vi "rotation_to_euler.vi"(11 "Rotation":T1) -> (3 "Theta XYZ":dbl[](array[numeric]))   [LabVIEW 2013]
uses:
  <vilib>/Analysis/Matrix/Datatypes/RealMatrix.ctl
  <vilib>/Analysis/Matrix/NI_Matrix.lvlib
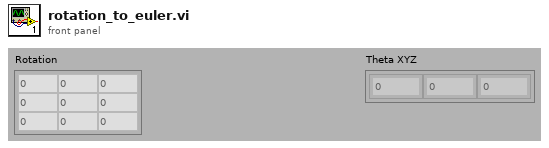
[diagram p1: front panel]
types:
  T1 = typedef "NI_Matrix.lvlib/RealMatrix.ctl" = dbl[][]
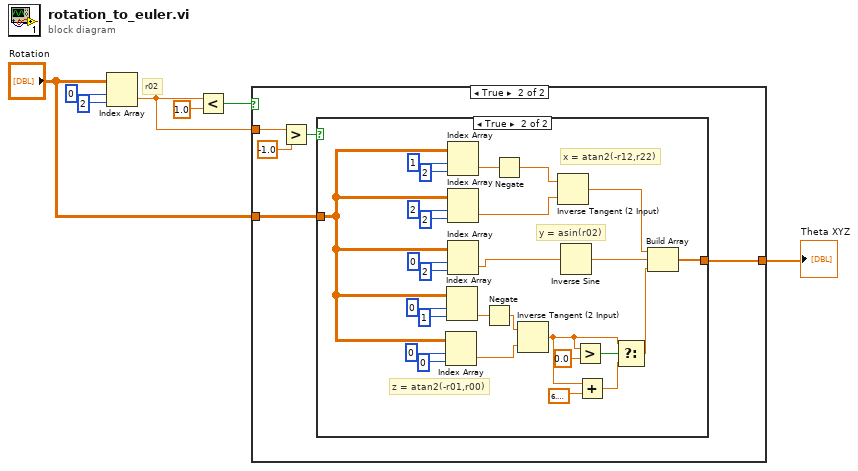
[diagram p0: block diagram]
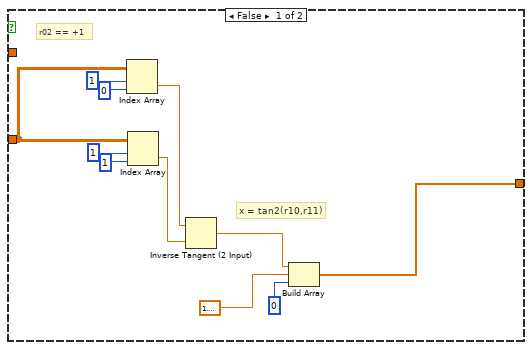
[diagram p2: hidden frame]
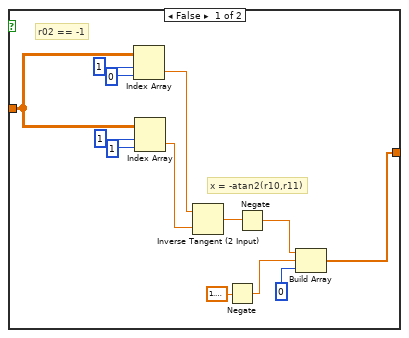
[diagram p3: hidden frame]
diagram:
  # "r02"
  n1 = Index Array(array="Rotation", index (row)=0, index (col)=2) -> (element=w3:dbl)
  n2 = Less?(x=w3, y=1.0) -> (x < y?=w5:bool)
  n3 = case shown="True" w5 {
    tunnel: "Rotation" -> [w13 w20]
    tunnel: w3 -> [_ w23]
    tunnel: [w8 w19] -> w1
    frame False {
      # "x = tan2(r10,r11)"
      # "r02 == +1"
      n4 = Index Array(array=w13, index (row)=1, index (col)=0) -> (element=w10:dbl)
      n5 = Index Array(array=w13, index (row)=1, index (col)=1) -> (element=w11:dbl)
      n6 = Inverse Tangent (2 Input)(1:w11, 2:w10) -> (0:w12:dbl)
      n7 = Build Array(w12, 1.5707963267948966, 0) -> (w8:dbl[])
    }
    frame True {
      n8 = Greater?(x=w23, y=-1.0) -> (0:w21:bool)
      n9 = case shown="True" w21 {
        tunnel: w20 -> [w27 w53]
        tunnel: [w24 w43] -> w19
        frame False {
          # "x = -atan2(r10,r11)"
          # "r02 == -1"
          n10 = Index Array(array=w27, index (row)=1, index (col)=0) -> (element=w28:dbl)
          n11 = Index Array(array=w27, index (row)=1, index (col)=1) -> (element=w29:dbl)
          n12 = Inverse Tangent (2 Input)(1:w29, 2:w28) -> (0:w26:dbl)
          n13 = Negate(x=1.5707963267948966) -> (-x=w30:dbl)
          n14 = Negate(x=w26) -> (-x=w25:dbl)
          n15 = Build Array(w25, w30, 0) -> (w24:dbl[])
        }
        frame True {
          # "z = atan2(-r01,r00)"
          # "x = atan2(-r12,r22)"
          # "y = asin(r02)"
          n16 = Index Array(array=w53, index (row)=0, index (col)=0) -> (element=w47:dbl)
          n17 = Index Array(array=w53, index (row)=0, index (col)=1) -> (element=w49:dbl)
          n18 = Index Array(array=w53, index (row)=1, index (col)=2) -> (element=w52:dbl)
          n19 = Index Array(array=w53, index (row)=2, index (col)=2) -> (element=w50:dbl)
          n20 = Index Array(array=w53, index (row)=0, index (col)=2) -> (element=w46:dbl)
          n21 = Negate(x=w49) -> (-x=w48:dbl)
          n22 = Negate(x=w52) -> (-x=w51:dbl)
          n23 = Inverse Tangent (2 Input)(1:w47, 2:w48) -> (0:w39:dbl)
          n24 = Inverse Tangent (2 Input)(1:w50, 2:w51) -> (0:w45:dbl)
          n25 = Inverse Sine(1:w46) -> (0:w44:dbl)
          n26 = Greater?(x=w39, y=0.0) -> (0:w40:bool)
          n27 = Add(x=w39, y=6.283185307179586) -> (x+y=w38:dbl)
          n28 = Select(t=w39, s=w40, f=w38) -> (s? t:f=w37:dbl)
          n29 = Build Array(w45, w44, w37) -> (w43:dbl[])
        }
      }
    }
  }
  "Theta XYZ" <- w1
